vi "Test String Length.vi"(8 "error in (no error)":errorcluster) -> (0 "error out":errorcluster, 3 "Pass?":bool)   [LabVIEW 2020]
uses:
  G-Unicode/Types/UTF-8 String/UTF-8 String.lvclass/UTF-8 String.ctl
  afc09de1-d9a4-4e26-9d52-ac1d88bb7c1d.vi
  b0f689db-263b-41ba-8052-3b219af6c750.vi
  afc09de1-d9a4-4e26-9d52-ac1d88bb7c1d.vi/48befa68-7cf9-4ae3-99f1-d639aefecf6e.vi
  b0f689db-263b-41ba-8052-3b219af6c750.vi/48befa68-7cf9-4ae3-99f1-d639aefecf6e.vi
  G-Unicode/Types/UTF-8 String/Read Encoded UTF-8 String.vi
  G-Unicode/Types/UTF-8 String/UTF-8 String.lvclass
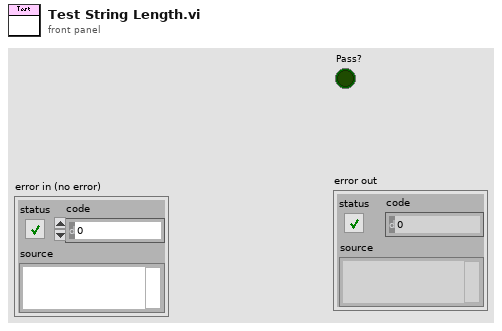
[diagram p1: front panel]
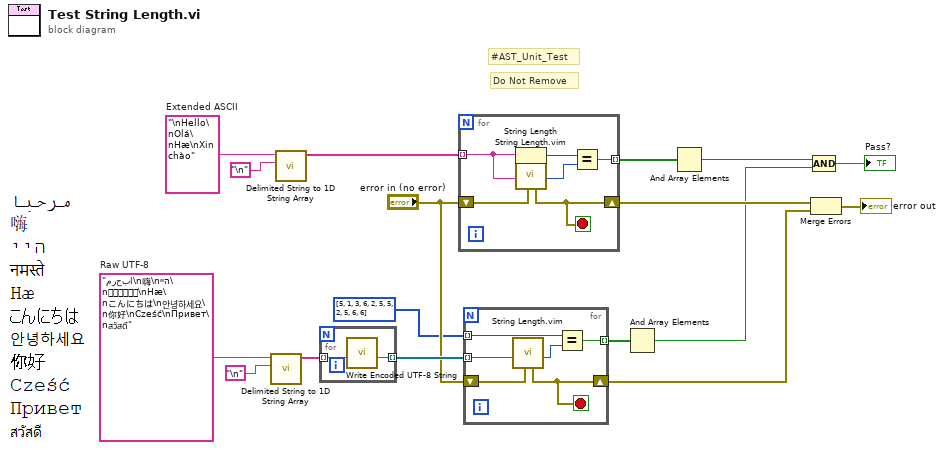
[diagram p0: block diagram]
diagram:
  w3 = "\nHello\nOlá\nHæ\nXin chào"  # Extended ASCII
  w16 = "مرحبا\n嗨\nהיי\nनमस्ते\nHæ\nこんにちは\n안녕하세요\n你好\nCześć\nПривет\nสวัสดี"  # Raw UTF-8
  # "Do Not Remove"
  # "#AST_Unit_Test"
  n1 = call <vilib>:"Delimited String to 1D String Array.vi"("delimiter"="\n", "delimited string"=w16) -> ("string array"=w15:string[])  [unwired: 9 in]
  n2 = call <vilib>:"Delimited String to 1D String Array.vi"("delimiter"="\n", "delimited string"=w3) -> ("string array"=w2:string[])  [unwired: 9 in]
  n3 = for {
    tunnel: w15 -> [w19] mode=indexing
    tunnel: [w18] -> w6 mode=indexing
    n4 = call "Write Encoded UTF-8 String.vi"("Encoded UTF-8 String"=w19) -> ("UTF-8 String"=w18:refnum<class "UTF-8 String.lvclass">)  [unwired: 10 in]
  }
  n5 = for {
    tunnel: [w25] -> w11 mode=indexing
    shift-right: [w20] -> w14
    shift-left: "error in (no error)" -> [w21]
    tunnel: w2 -> [w22] mode=indexing
    stop <- w20 stop-if-true
    n6 = String Length(string=w22) -> (length=w24:i32)
    n7 = call "String Length.vim"("error in"=w21, "String"=w22) -> ("Length"=w23:i32, "error out"=w20:errorcluster)  [unwired: 8 in]
    n8 = Equal?(x=w24, y=w23) -> (x = y?=w25:bool)
  }
  n9 = for {
    tunnel: w6 -> [w30] mode=indexing
    tunnel: [w31] -> w9 mode=indexing
    shift-right: [w28] -> w7
    shift-left: "error in (no error)" -> [w29]
    tunnel: i32[] [5, 1, 3, 6, 2, 5, 5, 2, 5, 6, 6] ("Array") -> [w27] mode=indexing
    stop <- w28 stop-if-true
    n10 = call "String Length.vim"("error in"=w29, "String"=w30) -> ("Length"=w26:i32, "error out"=w28:errorcluster)  [unwired: 8 in]
    n11 = Equal?(x=w27, y=w26) -> (x = y?=w31:bool)
  }
  n12 = And Array Elements(Boolean array=w9) -> (logical AND=w8:bool)
  n13 = And Array Elements(Boolean array=w11) -> (logical AND=w10:bool)
  n14 = Merge Errors(w14, w7) -> (→"error out":errorcluster)
  n15 = Compound Arithmetic op=AND(w10, w8) -> (→"Pass?":bool)
